vi "SeCrTs-UI Commands_R.vi"(11 "Data FIFO Ref":T1) -> ()   [LabVIEW 2022 SP3]
doc: "Use this template to build a simple state machine design pattern. Each state executes code and determines which state to transition to."
uses:
  RT Controls/SeCrTs-Data FIFO.ctl
  RT Controls/SeCrTs-NS Enum.ctl
  RT Controls/SeCrTs-Data Type Control screen.ctl
  RT Controls/ATF Storage Haelth.ctl
  RT Support/SeCrTs-RT_Global_R.vi
panel:
  out "Sts":bool
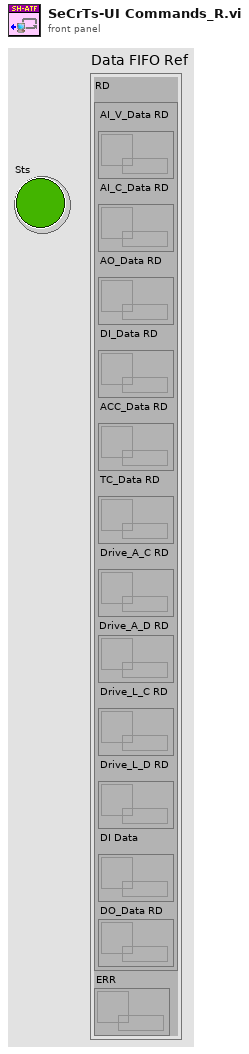
[diagram p1: front panel]
types:
  T1 = typedef "SeCrTs-Data FIFO.ctl" = cluster{"RD":cluster{"AI_V_Data RD":refnum<queue>, "AI_C_Data RD":refnum<queue>, "AO_Data RD":refnum<queue>, "DI_Data RD":refnum<queue>, "ACC_Data RD":refnum<queue>, "TC_Data RD":refnum<queue>, "Drive_A_C RD":refnum<queue>, "Drive_A_D RD":refnum<queue>, "Drive_L_C RD":refnum<queue>, "Drive_L_D RD":refnum<queue>, "DI Data":refnum<queue>, "DO_Data RD":refnum<queue>}, "ERR":refnum<queue>}
  T2 = cluster{"Reader":refnum<k21>, "Writer":refnum<k21>, "Er":refnum<queue>}
  T3 = typedef "SeCrTs-NS Enum.ctl" = enum16{"Initialize", "Listen for UI Writer", "Send data", "Exit"}
  T4 = typedef "ATF Storage Haelth.ctl" = enum16{"AI C", "AI V", "AO", "DI", "DO", "TC", "ACC", "RT Str", "DR A"}
  T5 = enum16{"Init", "Read 'All'", "Read 'n'", "Read '1'", "Write '1'", "Write 'n'", "Write 'All'"}
  T6 = cluster{"Start DAQ":bool, "Stop DAQ":bool, "RT Stop":bool, "RT Exit":bool, "Start Seq":bool}
  T7 = typedef "SeCrTs-Data Type Control screen.ctl" = cluster{"DI_Data":digitalwaveform[], "Drive_A_C":waveform(dbl)[], "Drive_A_D":waveform(dbl)[], "Drive_L_C":waveform(dbl)[], "Drive_L_D":waveform(dbl)[], "Loop Status":bool[], "CDT Timer":dbl, "RT Error":cluster{"Error Code":string, "Error Source":string}, "DO":waveform(dbl)[], "SEQ Monitor":string[], "Device List":string}
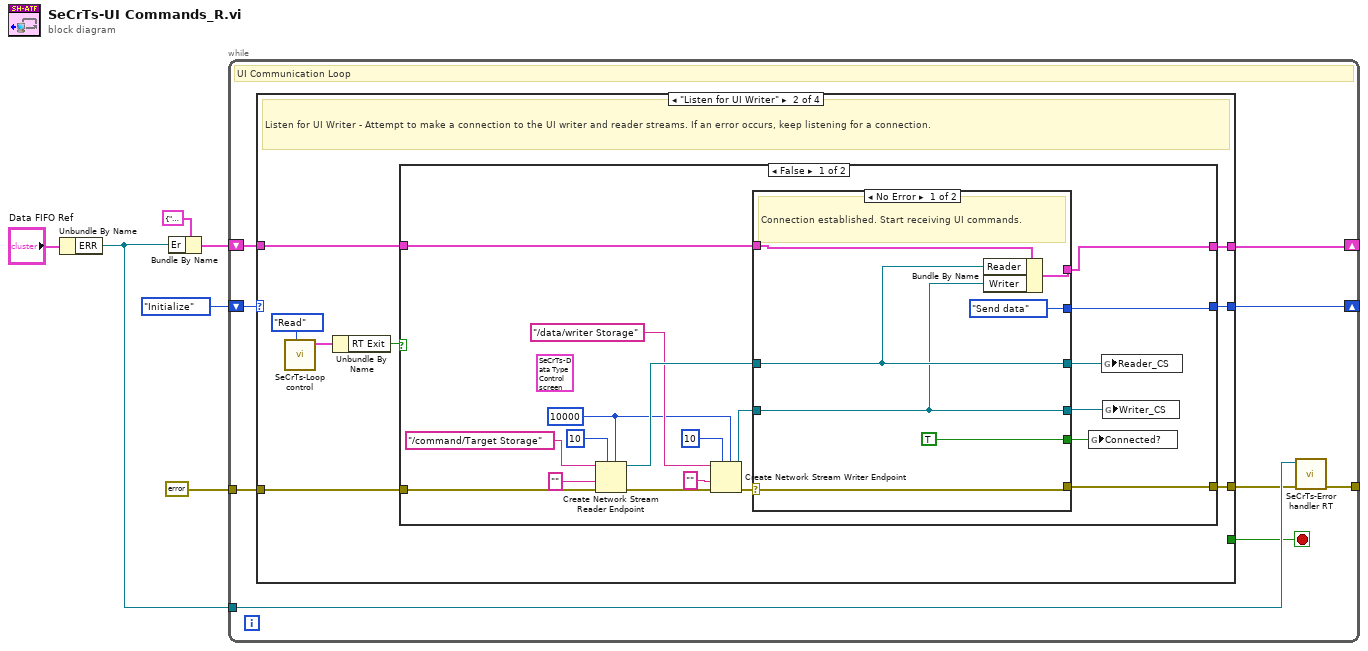
[diagram p0: block diagram]
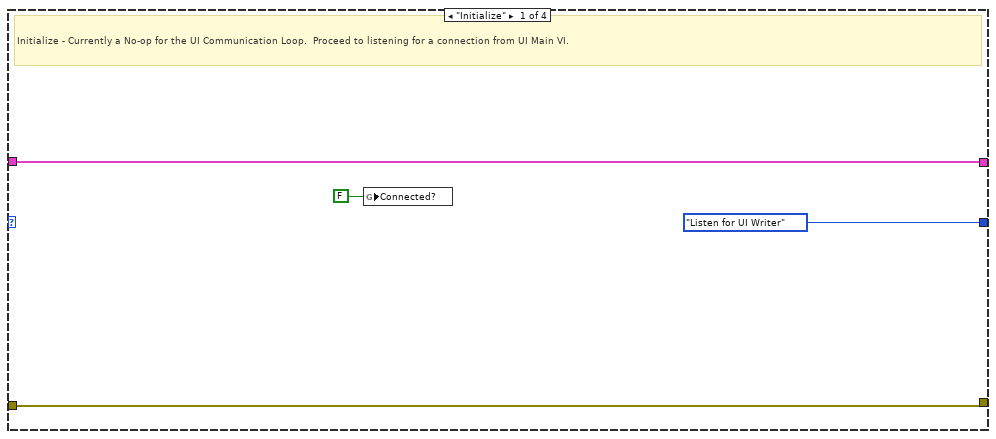
[diagram p2: hidden frame]
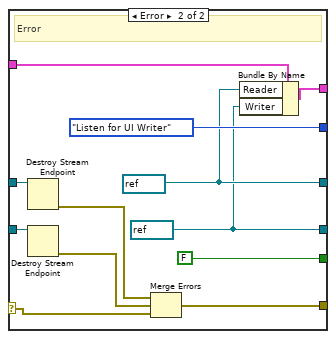
[diagram p3: hidden frame]
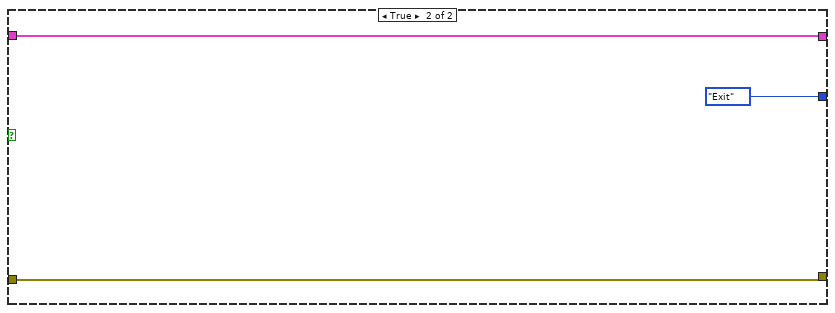
[diagram p4: hidden frame]
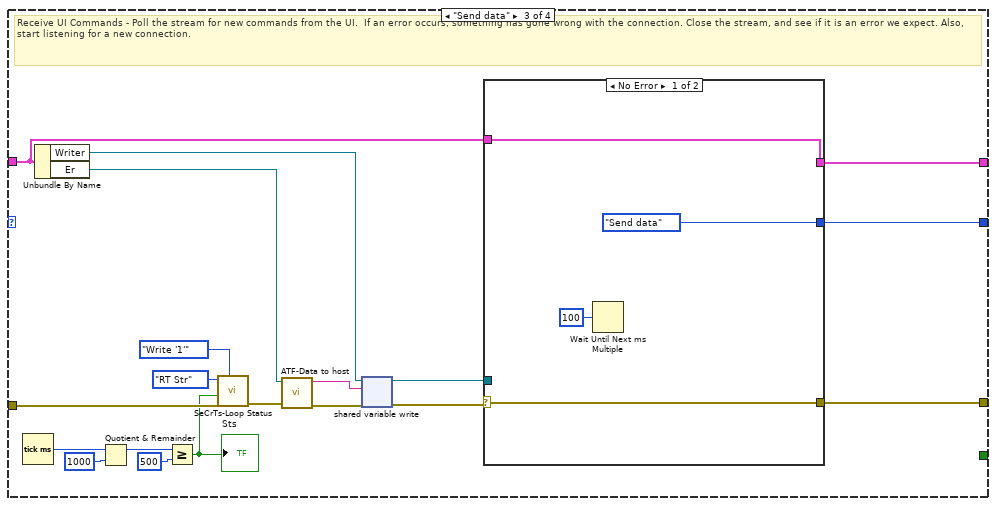
[diagram p5: hidden frame]
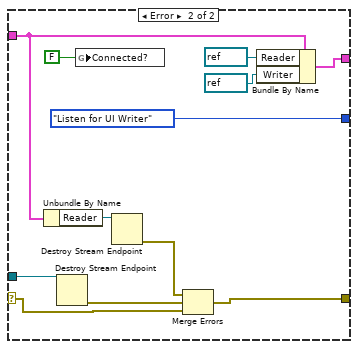
[diagram p6: hidden frame]
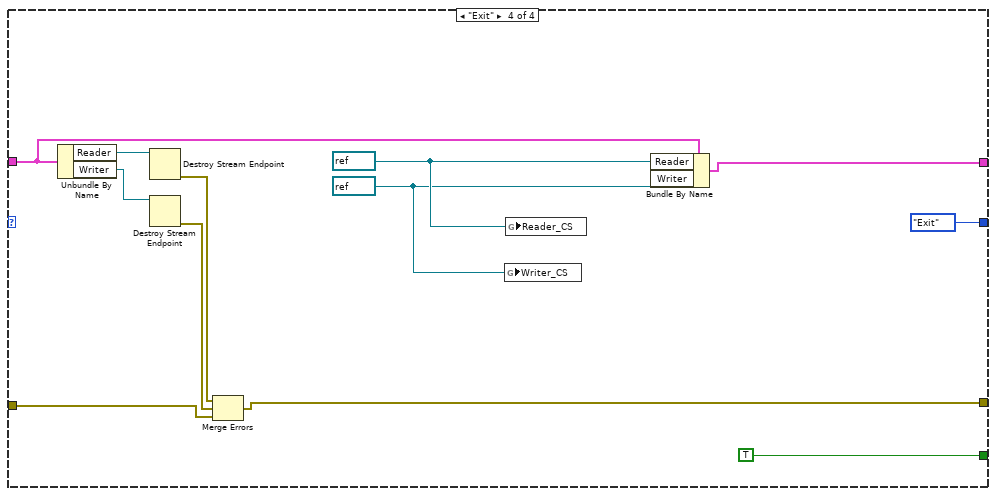
[diagram p7: hidden frame]
diagram:
  n1 = Unbundle By Name("Data FIFO Ref") -> ("ERR"=w1:refnum<queue>)
  n2 = Bundle By Name(cluster=T2 {"Reader"="", "Writer"="", "Er"=refnum}, "Er"=w1) -> (w4:T2)
  n3 = while {
    shift-right: [w14] -> _
    shift-left: SeCrTs-NS_Enum."Initialize" ("Enum") -> [w15]
    tunnel: w1 -> [w13]
    shift-right: [w9] -> _
    shift-left: w4 -> [w10]
    tunnel: errorcluster {"status"=FALSE, "code"=0, "source"=""} ("error in (no error)") -> [w11]
    tunnel: [w7] -> _
    stop <- w8 stop-if-true
    # "UI Communication Loop"
    n4 = case shown="\"Listen for UI Writer\"" w15 {
      tunnel: [w17 w27 w82 w113] -> w12
      tunnel: [SeCrTs-NS_Enum."Listen for UI Writer" ("Enum") w26 w83 SeCrTs-NS_Enum."Exit" ("Enum")] -> w14
      tunnel: w11 -> [w17 w25 w73 w104]
      tunnel: w10 -> [w16 w21 w79 w108]
      tunnel: [w16 w20 w80 w109] -> w9
      tunnel: [_ _ _ TRUE] -> w8
      frame "Initialize" {
        # "Initialize - Currently a No-op for the UI Communication Loop.  Proceed to listening for a connection from UI Main VI."
        n5 = global write "SeCrTs-RT_Global_R.vi" "Connected?"(FALSE ("Connected?")) -> ()
      }
      frame "Listen for UI Writer" {
        # "Listen for UI Writer - Attempt to make a connection to the UI writer and reader streams. If an error occurs, keep listening for a connection."
        n6 = call "SeCrTs-Loop control.vi"("Action"=enum16{"Init", "Write", "Read"}."Read") -> ("Loop Control out"=w23:T6)  [unwired: 9 in, 1 out]
        n7 = Unbundle By Name(w23) -> ("RT Exit"=w22:bool)
        n8 = case shown="False" w22 {
          tunnel: [w31 w66] -> w27
          tunnel: [w40 SeCrTs-NS_Enum."Exit" ("Enum")] -> w26
          tunnel: w25 -> [w34 w66]
          tunnel: w21 -> [w33 w67]
          tunnel: [w32 w67] -> w20
          frame False {
            w30 = 10000 ("timeout in ms (-1)")
            (unwired) T7 {"DI_Data"=[], "Drive_A_C"=[], "Drive_A_D"=[], "Drive_L_C"=[], "Drive_L_D"=[], "Loop Status"=[], "CDT Timer"=0.0, "RT Error"={"Error Code"="", "Error Source"=""}, "DO"=[], "SEQ Monitor"=[], "Device List"=""}
            n9 = Create Network Stream Reader Endpoint(5:w30, 7:10 ("reader buffer size"), 8:w34, 9:"" ("writer url"), 11:"/command/Target Storage" ("reader name")) -> (0:w45:errorcluster, 3:w46:refnum<k21>)  [unwired: 2 in]
            n10 = Create Network Stream Writer Endpoint(5:w30, 7:10 ("writer buffer size"), 8:w45, 9:"" ("reader url"), 11:"/data/writer Storage" ("RT Stream Name_C")) -> (0:w43:errorcluster, 3:w44:refnum<k21>)  [unwired: 2 in]
            n11 = case shown="No Error" w43 {
              selector: w43 -> [w47 w57]
              tunnel: w46 -> [w49 w65]
              tunnel: w44 -> [w48 w64]
              tunnel: [w49 w55] -> w39
              tunnel: [SeCrTs-NS_Enum."Send data" ("Enum") SeCrTs-NS_Enum."Listen for UI Writer" ("Enum")] -> w40
              tunnel: [w48 w54] -> w38
              tunnel: [TRUE ("Connected?") FALSE ("Connected?")] -> w35
              tunnel: w33 -> [w51 w61]
              tunnel: [w50 w60] -> w32
              tunnel: [w47 w56] -> w31
              frame No Error {
                # "Connection established. Start receiving UI commands."
                n12 = Bundle By Name(cluster=w51, "Reader"=w49, "Writer"=w48) -> (w50:T2)
              }
              frame Error {
                w54 = refnum<k21> refnum ("RT Stream Name_C")
                w55 = refnum<k21> refnum ("reader name")
                # "Error"
                n13 = Destroy Stream Endpoint(11:w65) -> (0:w59:errorcluster)  [unwired: 1 in]
                n14 = Destroy Stream Endpoint(11:w64) -> (0:w58:errorcluster)  [unwired: 1 in]
                n15 = Merge Errors(w59, w58, w57) -> (w56:errorcluster)
                n16 = Bundle By Name(cluster=w61, "Reader"=w55, "Writer"=w54) -> (w60:T2)
              }
            }
            n17 = global write "SeCrTs-RT_Global_R.vi" "Connected?"(w35) -> ()
            n18 = global write "SeCrTs-RT_Global_R.vi" "Reader_CS"(w39) -> ()
            n19 = global write "SeCrTs-RT_Global_R.vi" "Writer_CS"(w38) -> ()
          }
          frame True {
          }
        }
      }
      frame "Send data" {
        # "Receive UI Commands - Poll the stream for new commands from the UI.  If an error occurs, something has gone wrong with the connection. Close the stream, and see if it is an error we expect. Also, start listening for a new connection."
        n20 = Tick Count (ms)() -> (millisecond timer value=w77:u32)
        n21 = Unbundle By Name(w79) -> ("Writer"=w86:refnum<k21>, "Er"=w85:refnum<queue>)
        n22 = Quotient & Remainder(x=w77, y=u32 1000) -> (x-y*floor(x/y)=w74:u32)  [unwired: 1 out]
        n23 = Greater Or Equal?(x=w74, y=u32 500) -> (x >= y?=w69:bool)
        "Sts" <- w69
        n24 = call "SeCrTs-Loop Status.vi"("Option"=T5."Write '1'", "error in (no error)"=w73, "Status"=w69, "Loop"=ATF_Storage_Haelth."RT Str") -> ("error out"=w72:errorcluster)  [unwired: 5 in, 2 out]
        n25 = call "ATF-Data to host.vi"("error in (no error)"=w72, "Err"=w85) -> ("error out"=w87:errorcluster, "Data"=w78:string)  [unwired: 8 in]
        n26 = shared-variable-write(w86, w87, w78) -> (w81:refnum<k21>, w84:errorcluster)  [unwired: 1 in, 1 out]
        n27 = case shown="No Error" w84 {
          selector: w84 -> [w89 w99]
          tunnel: [SeCrTs-NS_Enum."Send data" ("Enum") SeCrTs-NS_Enum."Listen for UI Writer" ("Enum")] -> w83
          tunnel: [w89 w102] -> w82
          tunnel: w81 -> [_ w98]
          tunnel: [w88 w95] -> w80
          tunnel: w79 -> [w88 w94]
          frame No Error {
            n28 = Wait Until Next ms Multiple(millisecond multiple=u32 100) -> ()  [unwired: 1 out]
          }
          frame Error {
            n29 = Unbundle By Name(w94) -> ("Reader"=w97:refnum<k21>)
            n30 = Destroy Stream Endpoint(11:w98) -> (0:w100:errorcluster)  [unwired: 1 in]
            n31 = global write "SeCrTs-RT_Global_R.vi" "Connected?"(FALSE ("Connected?")) -> ()
            n32 = Destroy Stream Endpoint(11:w97) -> (0:w101:errorcluster)  [unwired: 1 in]
            n33 = Merge Errors(w101, w100, w99) -> (w102:errorcluster)
            n34 = Bundle By Name(cluster=w94, "Reader"=refnum<k21> refnum, "Writer"=refnum<k21> refnum) -> (w95:T2)
          }
        }
      }
      frame "Exit" {
        w105 = refnum<k21> refnum ("Writer")
        w106 = refnum<k21> refnum ("Reader")
        n35 = Unbundle By Name(w108) -> ("Reader"=w115:refnum<k21>, "Writer"=w114:refnum<k21>)
        n36 = Destroy Stream Endpoint(11:w115) -> (0:w112:errorcluster)  [unwired: 1 in]
        n37 = Destroy Stream Endpoint(11:w114) -> (0:w111:errorcluster)  [unwired: 1 in]
        n38 = Merge Errors(w112, w111, w104) -> (w113:errorcluster)
        n39 = global write "SeCrTs-RT_Global_R.vi" "Writer_CS"(w105) -> ()
        n40 = global write "SeCrTs-RT_Global_R.vi" "Reader_CS"(w106) -> ()
        n41 = Bundle By Name(cluster=w108, "Reader"=w106, "Writer"=w105) -> (w109:T2)
      }
    }
    n42 = call "SeCrTs-Error handler RT.vi"("error in"=w12, "Message Queue"=w13) -> ("error out"=w7:errorcluster)  [unwired: 8 in, 1 out]
  }
